vi "CleanUp.vi"(8 "error in (no error)":errorcluster, 11 "reference in":refnum<class "Static TestSuite.lvclass">) -> (0 "error out":errorcluster, 3 "reference out":refnum<class "Static TestSuite.lvclass">)   [LabVIEW 2013, in "Static TestSuite.lvclass"]
uses:
  Static TestSuite.lvclass
  Classes/TestSuite/TestSuite.lvclass
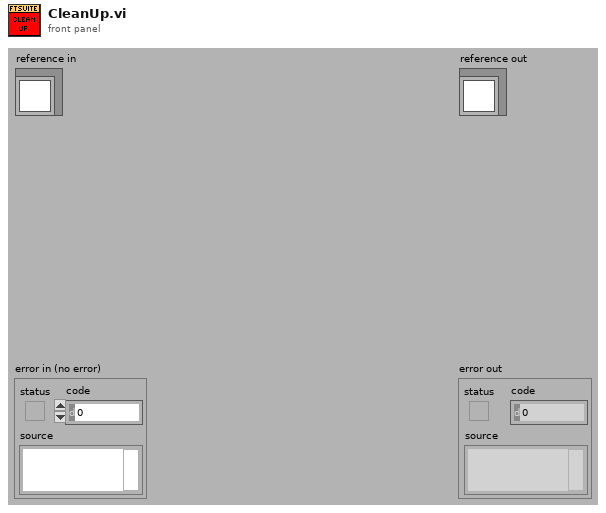
[diagram p1: front panel]
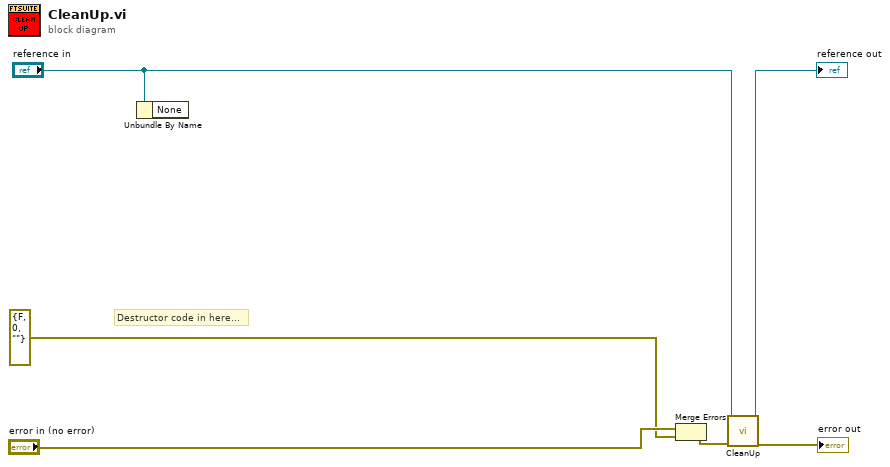
[diagram p0: block diagram]
diagram:
  # "Destructor code in here..."
  n1 = Unbundle By Name("reference in") -> ()  [unwired: 1 out]
  n2 = Merge Errors("error in (no error)", errorcluster {"status"=FALSE, "code"=0, "source"=""} ("error in (no error)")) -> (w2:errorcluster)
  n3 = call-parent "CleanUp.vi"("error in (no error)"=w2, "TestSuite in"="reference in") -> ("error out"=→"error out":errorcluster, "TestSuite out"=→"reference out":refnum<class "Static TestSuite.lvclass">)  [unwired: 8 in]
